vi "AMZ_S3_ERR_Create Error Cluster from Response body.vi"(8 "error in (no error)":errorcluster, 11 "Response body":string) -> (0 "error out":errorcluster, 3 "Is Throttled?":bool)   [LabVIEW 2015, in "LV Interface for Amazon S3.lvlib"]
uses:
  LV Interface for Amazon S3.lvlib
  XML Parser/XML Parser.lvlib
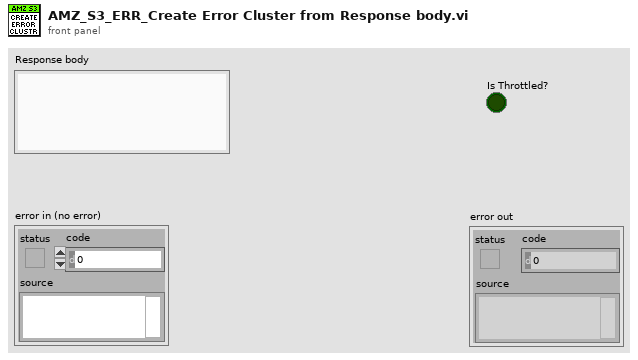
[diagram p1: front panel]
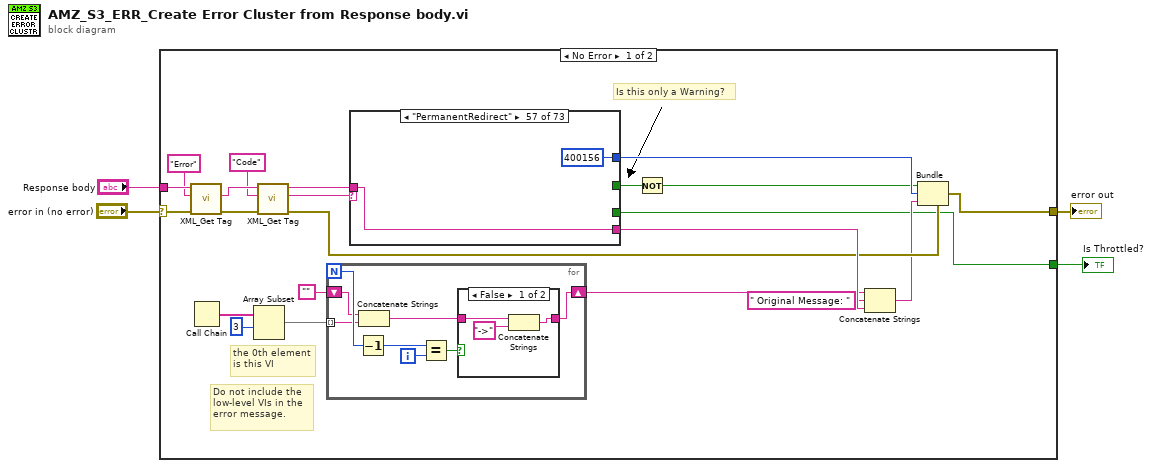
[diagram p0: block diagram]
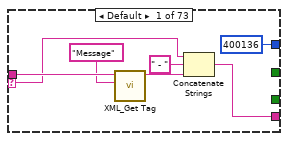
[diagram p3: hidden frame]
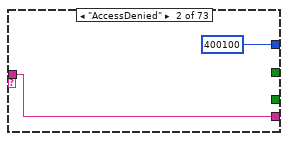
[diagram p4: hidden frame]
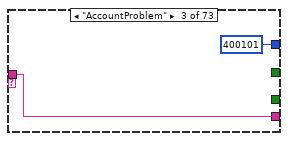
[diagram p5: hidden frame]
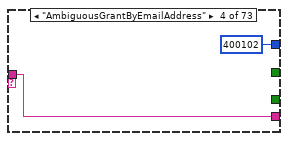
[diagram p6: hidden frame]
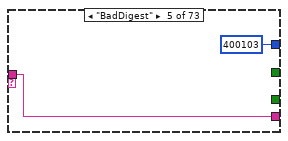
[diagram p7: hidden frame]
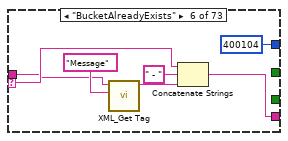
[diagram p8: hidden frame]
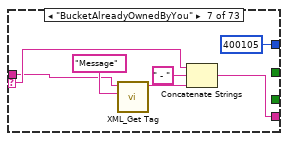
[diagram p9: hidden frame]
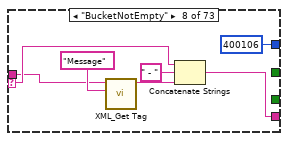
[diagram p10: hidden frame]
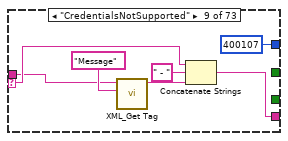
[diagram p11: hidden frame]
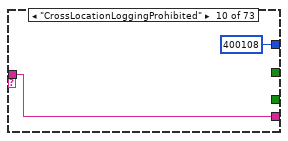
[diagram p12: hidden frame]
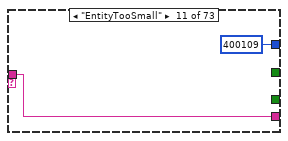
[diagram p13: hidden frame]
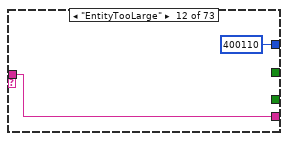
[diagram p14: hidden frame]
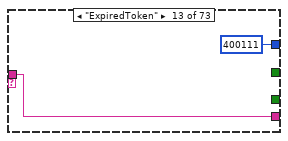
[diagram p15: hidden frame]
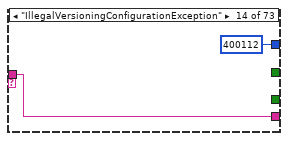
[diagram p16: hidden frame]
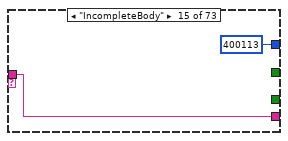
[diagram p17: hidden frame]
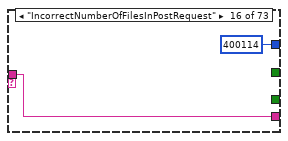
[diagram p18: hidden frame]
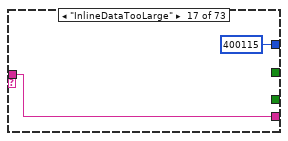
[diagram p19: hidden frame]
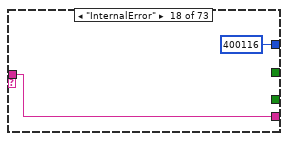
[diagram p20: hidden frame]
diagram:
  n1 = case shown="No Error" "error in (no error)" {
    selector: "error in (no error)" -> [w19 w214]
    tunnel: "Response body" -> [w26 _]
    tunnel: [w9 w214] -> w3
    tunnel: [w5 FALSE] -> w1
    frame No Error {
      # "Do not include the\nlow-level VIs in the\nerror message."
      # "Is this only a Warning?"
      # "the 0th element\nis this VI"
      n2 = call "XML_Get Tag.vi"("error in (no error)"=w19, "Tag name"="Error", "XML String in"=w26) -> ("error out"=w24:errorcluster, "Tag value"=w23:string)  [unwired: 4 in, 3 out]
      n3 = Call Chain() -> (call chain=w17:string[])
      n4 = Array Subset(array=w17, index=3) -> (w15:string[])  [unwired: 1 in]
      n5 = call "XML_Get Tag.vi"("error in (no error)"=w24, "Tag name"="Code", "XML String in"=w23) -> ("error out"=w12:errorcluster, "Tag value"=w21:string, "XML String dup"=w8:string)  [unwired: 4 in, 2 out]
      n6 = for {
        N -> [w31]
        tunnel: w15 -> [w29] mode=indexing
        shift-right: [w27] -> w13
        shift-left: "" -> [w30]
        i -> [w28]
        n7 = Decrement(x=w31) -> (x-1=w34:i32)
        n8 = Concatenate Strings(w30, w29) -> (w32:string)
        n9 = Equal?(x=w34, y=w28) -> (x = y?=w33:bool)
        n10 = case shown="False" w33 {
          tunnel: w32 -> [w37 w38]
          tunnel: [w35 w38] -> w27
          frame False {
            n11 = Concatenate Strings(w37, "->" ("Substring")) -> (w35:string)
          }
          frame True {
          }
        }
      }
      n12 = case shown="\"PermanentRedirect\"" w21 {
        selector: w21 -> [w41 _ _ _ _ w55 w63 w70 w76 _ _ _ _ _ _ _ _ _ _ _ _ _ _ _ _ _ _ _ _ _ _ _ _ _ _ _ _ _ _ _ _ _ _ _ _ _ _ _ _ _ _ _ _ _ _ _ _ _ _ _ _ _ _ _ _ _ _ _ _ _ _ _ _]
        tunnel: [400136 400100 400101 400102 400103 400104 400105 400106 400107 400108 400109 400110 400111 400112 400113 400114 400115 400116 400117 400118 400119 400120 400121 400122 400123 400124 400125 400126 400127 400128 400129 400130 400131 400132 400133 400134 400135 400137 400138 400139 400140 400141 400142 400143 400144 400145 400146 400147 400148 400149 400150 400151 400152 400153 400154 400155 400156 400157 400158 400159 400160 400161 400162 400163 400164 400165 1 400166 400167 400168 400169 400170 400171] -> w11
        tunnel: [_ _ _ _ _ _ _ _ _ _ _ _ _ _ _ _ _ _ _ _ _ _ _ _ _ _ _ _ _ _ _ _ _ _ _ _ _ _ _ _ _ _ _ _ _ _ _ _ _ _ _ _ _ _ _ _ _ _ TRUE _ _ _ _ _ _ TRUE w199 _ _ _ _ _ _] -> w20
        tunnel: w8 -> [w44 w46 w48 w50 w52 w54 w62 w69 w75 w82 w84 w86 w88 w90 w92 w94 w96 w98 w100 w102 w104 w106 w108 w110 w112 w114 w116 w118 w120 w122 w124 w126 w128 w130 w132 w134 w136 w138 w140 w142 w144 w146 w148 w150 w152 w154 w156 w158 w160 w162 w164 w166 w168 w170 w172 w174 w176 w178 w180 w183 w185 w187 w189 w191 w193 w195 w200 w201 w203 w205 w207 w209 w211]
        tunnel: [w39 w46 w48 w50 w52 w56 w61 w68 w77 w82 w84 w86 w88 w90 w92 w94 w96 w98 w100 w102 w104 w106 w108 w110 w112 w114 w116 w118 w120 w122 w124 w126 w128 w130 w132 w134 w136 w138 w140 w142 w144 w146 w148 w150 w152 w154 w156 w158 w160 w162 w164 w166 w168 w170 w172 w174 w176 w178 w180 w183 w185 w187 w189 w191 w193 w195 w200 w201 w203 w205 w207 w209 w211] -> w14
        tunnel: [_ _ _ _ _ _ _ _ _ _ _ _ _ _ _ _ _ _ _ _ _ _ _ _ _ _ _ _ _ _ _ _ _ _ _ _ _ _ _ _ _ _ _ _ _ _ _ _ _ _ _ _ _ _ _ _ _ _ _ _ _ _ _ _ _ _ w199 _ _ _ _ _ _] -> w5
        frame Default {
          n13 = call "XML_Get Tag.vi"("Tag name"="Message", "XML String in"=w44) -> ("XML String dup"=w42:string)  [unwired: 5 in, 4 out]
          n14 = Concatenate Strings(w41, " - " ("string"), w42) -> (w39:string)
        }
        frame "AccessDenied" {
        }
        frame "AccountProblem" {
        }
        frame "AmbiguousGrantByEmailAddress" {
        }
        frame "BadDigest" {
        }
        frame "BucketAlreadyExists" {
          n15 = call "XML_Get Tag.vi"("Tag name"="Message", "XML String in"=w54) -> ("XML String dup"=w58:string)  [unwired: 5 in, 4 out]
          n16 = Concatenate Strings(w55, " - " ("string"), w58) -> (w56:string)
        }
        frame "BucketAlreadyOwnedByYou" {
          n17 = call "XML_Get Tag.vi"("Tag name"="Message", "XML String in"=w62) -> ("XML String dup"=w65:string)  [unwired: 5 in, 4 out]
          n18 = Concatenate Strings(w63, " - " ("string"), w65) -> (w61:string)
        }
        frame "BucketNotEmpty" {
          n19 = call "XML_Get Tag.vi"("Tag name"="Message", "XML String in"=w69) -> ("XML String dup"=w72:string)  [unwired: 5 in, 4 out]
          n20 = Concatenate Strings(w70, " - " ("string"), w72) -> (w68:string)
        }
        frame "CredentialsNotSupported" {
          n21 = call "XML_Get Tag.vi"("Tag name"="Message", "XML String in"=w75) -> ("XML String dup"=w79:string)  [unwired: 5 in, 4 out]
          n22 = Concatenate Strings(w76, " - " ("string"), w79) -> (w77:string)
        }
        frame "CrossLocationLoggingProhibited" {
        }
        frame "EntityTooSmall" {
        }
        frame "EntityTooLarge" {
        }
        frame "ExpiredToken" {
        }
        frame "IllegalVersioningConfigurationException" {
        }
        frame "IncompleteBody" {
        }
        frame "IncorrectNumberOfFilesInPostRequest" {
        }
        frame "InlineDataTooLarge" {
        }
        frame "InternalError" {
        }
        frame "InvalidAccessKeyId" {
        }
        frame "InvalidAddressingHeader" {
        }
        frame "InvalidArgument" {
        }
        frame "InvalidBucketName" {
        }
        frame "InvalidDigest" {
        }
        frame "InvalidLocationConstraint" {
        }
        frame "InvalidPart" {
        }
        frame "InvalidPartOrder" {
        }
        frame "InvalidPayer" {
        }
        frame "InvalidPolicyDocument" {
        }
        frame "InvalidRange" {
        }
        frame "InvalidSecurity" {
        }
        frame "InvalidSOAPRequest" {
        }
        frame "InvalidStorageClass" {
        }
        frame "InvalidTargetBucketForLogging" {
        }
        frame "InvalidToken" {
        }
        frame "InvalidURI" {
        }
        frame "KeyTooLong" {
        }
        frame "MalformedACLError" {
        }
        frame "MalformedPOSTRequest" {
        }
        frame "MalformedXML" {
        }
        frame "MaxMessageLengthExceeded" {
        }
        frame "MaxPostPreDataLengthExceededError" {
        }
        frame "MetadataTooLarge" {
        }
        frame "MethodNotAllowed" {
        }
        frame "MissingAttachment" {
        }
        frame "MissingContentLength" {
        }
        frame "MissingRequestBodyError" {
        }
        frame "MissingSecurityElement" {
        }
        frame "MissingSecurityHeader" {
        }
        frame "NoLoggingStatusForKey" {
        }
        frame "NoSuchBucket" {
        }
        frame "NoSuchKey" {
        }
        frame "NoSuchUpload" {
        }
        frame "NoSuchVersion" {
        }
        frame "NotImplemented" {
        }
        frame "NotSignedUp" {
        }
        frame "OperationAborted" {
        }
        frame "PermanentRedirect" {
        }
        frame "PreconditionFailed" {
        }
        frame "Redirect" {
        }
        frame "RequestIsNotMultiPartContent" {
        }
        frame "RequestTimeout" {
        }
        frame "RequestTimeTooSkewed" {
        }
        frame "RequestTorrentOfBucketError" {
        }
        frame "SignatureDoesNotMatch" {
        }
        frame "SlowDown" {
        }
        frame "TemporaryRedirect" {
        }
        frame "Throttling" {
          w199 = TRUE
        }
        frame "TokenRefreshRequired" {
        }
        frame "TooManyBuckets" {
        }
        frame "UnexpectedContent" {
        }
        frame "UnresolvableGrantByEmailAddress" {
        }
        frame "UserKeyMustBeSpecified" {
        }
        frame "NoSuchBucketPolicy" {
        }
      }
      n23 = Not(x=w20) -> (.not. x?=w10:bool)
      n24 = Concatenate Strings(w13, " Original Message: " ("string"), w14) -> (w6:string)
      n25 = Bundle(cluster=w12, "status"=w10, "code"=w11, "source"=w6) -> (w9:errorcluster)
    }
    frame Error {
    }
  }
  "error out" <- w3
  "Is Throttled?" <- w1
